vi "Initialize Tree.vi"(8 "error in":errorcluster, 10 "reference":refnum<vi>, 11 "tdms file":refnum<k34>) -> (0 "error out":errorcluster, 2 "tree reference out":refnum<vi>, 3 "tdms file out":refnum<k34>)   [LabVIEW 2019, in "Report Viewer.lvlib" / "Report Viewer.lvclass"]
uses:
  Report Viewer.lvclass
panel:
  out "Group Load":u64(slide)=38 scale=-1.0..1260.0
  out "TDMS Load":u64(slide)=38 scale=-1.0..11.0
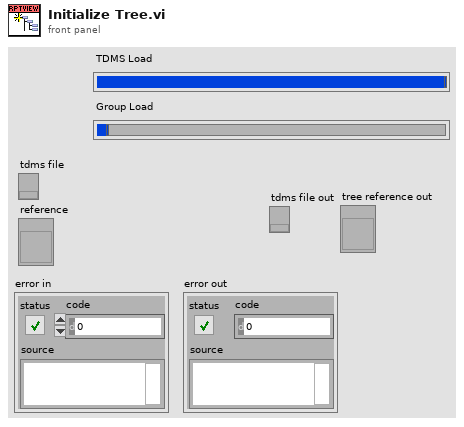
[diagram p1: front panel]
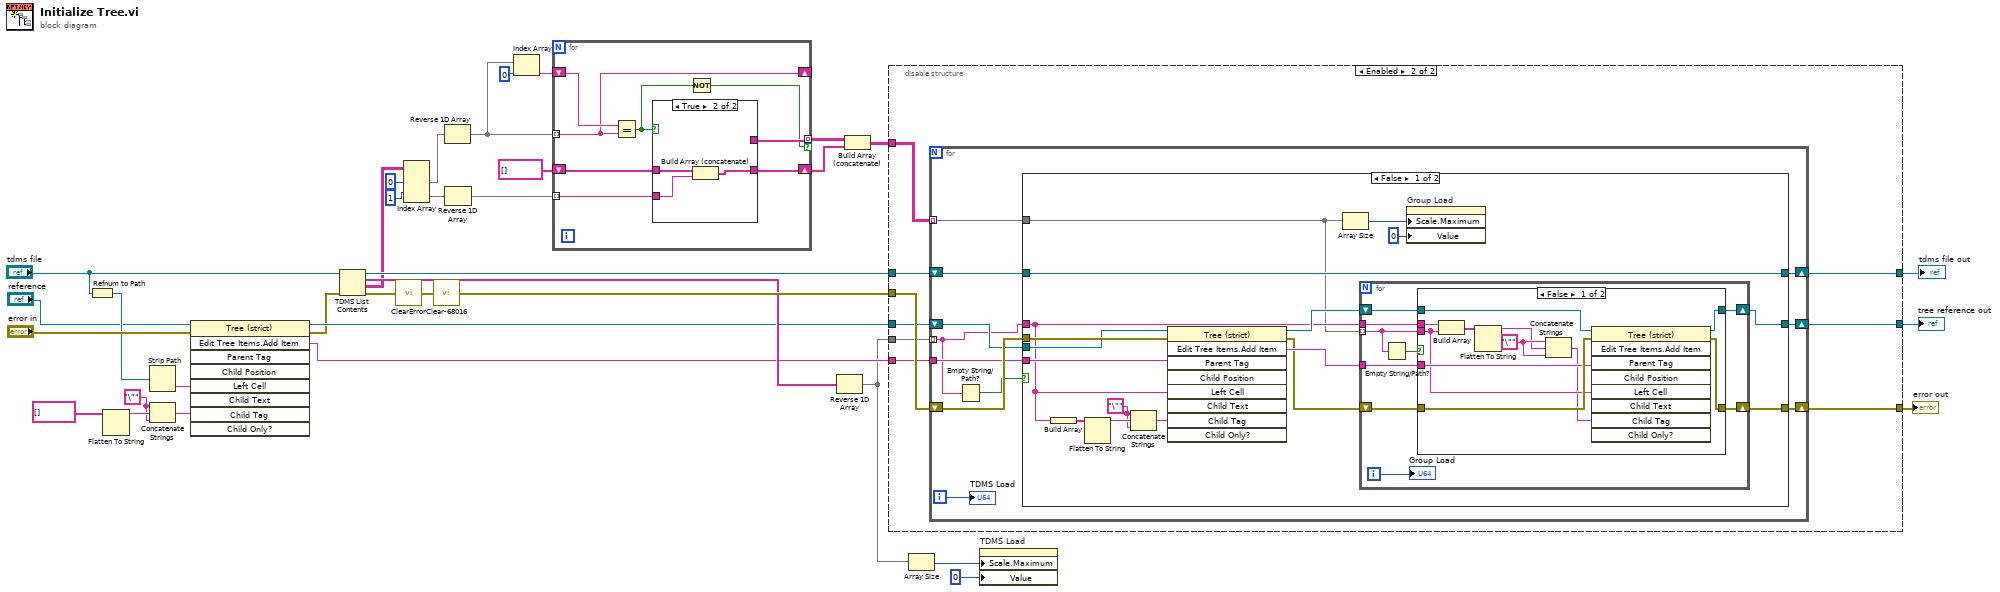
[diagram p0: block diagram]
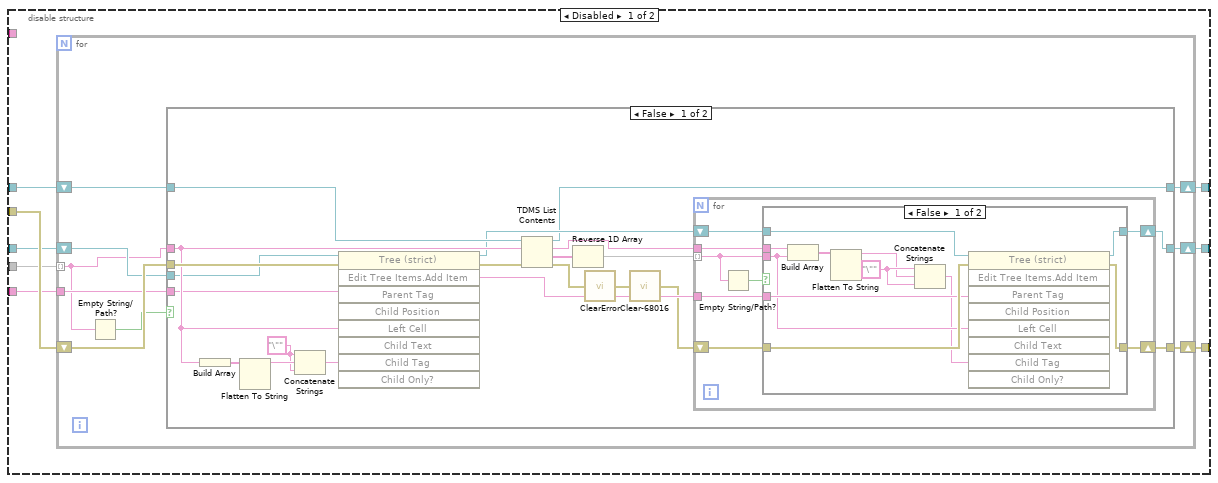
[diagram p2: hidden frame]
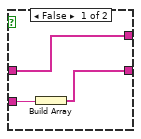
[diagram p7: hidden frame]
diagram:
  w28 = "\"" ("string")
  n1 = Refnum to Path(1:"tdms file") -> (0:w20:path)
  n2 = Flatten To String(anything=string[] [] ("appended array")) -> (data string=w29:string)  [unwired: 3 in, 2 out]
  n3 = Strip Path(path=w20) -> (name=w27:string)  [unwired: 1 out]
  n4 = Concatenate Strings(w28, w29, w28) -> (w31:string)
  n5 = invoke on="Invoke Node" class="Tree (strict)" method="Edit Tree Items.Add Item"(reference="reference", error in="error in", "Left Cell"=w27, "Child Tag"=w31) -> (reference out=w26:refnum<vi>, error out=w25:errorcluster, "Edit Tree Items:Add Item"=w32:string)  [unwired: 5 in, 6 out]
  n6 = TDMS List Contents(4:w25, 7:"tdms file") -> (0:w36:errorcluster, 1:w14:string[][], 2:w33:string[], 3:w24:refnum<k34>)  [unwired: 1 in]
  n7 = call <vilib>:"ClearError.vi"("error in (no error)"=w36) -> ("error out"=w34:errorcluster)
  n8 = Index Array(array=w14, index (row) #1=0 ("index (row)"), index (row) #2=1 ("index (row)")) -> (element #1=w2:string[], element #2=w1:string[])  [unwired: 2 in]
  n9 = call <vilib>:"Clear-68016.vi"("error in (no error)"=w34) -> ("error out"=w35:errorcluster)
  n10 = Reverse 1D Array(array=w2) -> (reversed array=w9:string[])
  n11 = Reverse 1D Array(array=w1) -> (reversed array=w12:string[])
  n12 = Index Array(array=w9, index=0) -> (element=w10:string)
  n13 = for {
    tunnel: w9 -> [w39] mode=indexing
    shift-right: [w39] -> _
    shift-left: w10 -> [w44]
    tunnel: w12 -> [w42] mode=indexing
    shift-right: [w37] -> w7
    shift-left: string[] [] -> [w43]
    tunnel: [w41] -> w8 mode=indexing if=w38
    n14 = Equal?(x=w44, y=w39) -> (x = y?=w40:bool)
    n15 = case shown="True" w40 {
      tunnel: w43 -> [w45 w49]
      tunnel: w42 -> [w46 w50]
      tunnel: [w47 w48] -> w37
      tunnel: [w45 _] -> w41
      frame False {
        n16 = Build Array(w46) -> (w47:string[])
      }
      frame True {
        n17 = Build Array (concatenate)(w49, w50) -> (w48:string[])
      }
    }
    n18 = Not(x=w40) -> (.not. x?=w38:bool)
  }
  n19 = Reverse 1D Array(array=w33) -> (reversed array=w21:string[])
  n20 = Build Array (concatenate)(w8, w7) -> (w6:string[][])
  n21 = disable-structure shown="Enabled" {
    disable-tunnel: w35 -> [w58 w121]
    disable-tunnel: w32 -> [w57 w120]
    disable-tunnel: w26 -> [w56 w119]
    disable-tunnel: w24 -> [w55 w118]
    disable-tunnel: [w54 w117] -> w23
    disable-tunnel: w21 -> [w53 w116]
    disable-tunnel: [w52 w115] -> w19
    disable-tunnel: [w51 w114] -> w18
    disable-tunnel: w6 -> [_ w113]
    frame Disabled {
      n22 = for {
        tunnel: w53 -> [w61] mode=indexing
        shift-right: [w64] -> w52
        shift-left: w55 -> [w66]
        shift-right: [w65] -> w54
        shift-left: w58 -> [w67]
        tunnel: w57 -> [w62]
        shift-right: [w59] -> w51
        shift-left: w56 -> [w63]
        n23 = Empty String/Path?(string/path=w61) -> (empty?=w60:bool)
        n24 = case shown="False" w60 {
          tunnel: w67 -> [w88 w111]
          tunnel: w66 -> [w86 w112]
          tunnel: [w85 w111] -> w65
          tunnel: [w70 w112] -> w64
          tunnel: w61 -> [w83 _]
          tunnel: w63 -> [w78 w110]
          tunnel: w62 -> [w76 _]
          tunnel: [w71 w110] -> w59
          frame False {
            w79 = "\"" ("string")
            n25 = Build Array(w83) -> (w82:string[])
            n26 = Flatten To String(anything=w82) -> (data string=w81:string)  [unwired: 3 in, 2 out]
            n27 = Concatenate Strings(w79, w81, w79) -> (w80:string)
            n28 = invoke on="Invoke Node" class="Tree (strict)" method="Edit Tree Items.Add Item"(reference=w78, error in=w88, "Parent Tag"=w76, "Left Cell"=w83, "Child Tag"=w80) -> (reference out=w77:refnum<vi>, error out=w87:errorcluster, "Edit Tree Items:Add Item"=w84:string)  [unwired: 4 in, 6 out]
            n29 = TDMS List Contents(4:w87, 6:w83, 7:w86) -> (0:w72:errorcluster, 1:w75:string[], 2:w69:string, 3:w70:refnum<k34>)
            n30 = Reverse 1D Array(array=w75) -> (reversed array=w68:string[])
            n31 = call <vilib>:"ClearError.vi"("error in (no error)"=w72) -> ("error out"=w74:errorcluster)
            n32 = call <vilib>:"Clear-68016.vi"("error in (no error)"=w74) -> ("error out"=w73:errorcluster)
            n33 = for {
              tunnel: w68 -> [w91] mode=indexing
              shift-right: [w95] -> w85
              shift-left: w73 -> [w96]
              tunnel: w84 -> [w94]
              tunnel: w69 -> [w93]
              shift-right: [w89] -> w71
              shift-left: w77 -> [w90]
              n34 = Empty String/Path?(string/path=w91) -> (empty?=w92:bool)
              n35 = case shown="False" w92 {
                tunnel: w96 -> [w107 w109]
                tunnel: [w106 w109] -> w95
                tunnel: w94 -> [w105 _]
                tunnel: w91 -> [w103 _]
                tunnel: w93 -> [w102 _]
                tunnel: w90 -> [w98 w108]
                tunnel: [w97 w108] -> w89
                frame False {
                  w101 = "\"" ("string")
                  n36 = Build Array(w102, w103) -> (w104:string[])
                  n37 = Flatten To String(anything=w104) -> (data string=w99:string)  [unwired: 3 in, 2 out]
                  n38 = Concatenate Strings(w101, w99, w101) -> (w100:string)
                  n39 = invoke on="Invoke Node" class="Tree (strict)" method="Edit Tree Items.Add Item"(reference=w98, error in=w107, "Parent Tag"=w105, "Left Cell"=w103, "Child Tag"=w100) -> (reference out=w97:refnum<vi>, error out=w106:errorcluster)  [unwired: 4 in, 7 out]
                }
                frame True {
                }
              }
            }
          }
          frame True {
          }
        }
      }
    }
    frame Enabled {
      n40 = for {
        tunnel: w116 -> [w126] mode=indexing
        shift-right: [w129] -> w115
        shift-left: w118 -> [w131]
        shift-right: [w130] -> w117
        shift-left: w121 -> [w132]
        tunnel: w120 -> [w127]
        shift-right: [w124] -> w114
        shift-left: w119 -> [w128]
        tunnel: w113 -> [w123] mode=indexing
        i -> [w122]
        n41 = Empty String/Path?(string/path=w126) -> (empty?=w125:bool)
        n42 = case shown="False" w125 {
          tunnel: w132 -> [w149 w173]
          tunnel: w131 -> [w136 w174]
          tunnel: [w148 w173] -> w130
          tunnel: [w136 w174] -> w129
          tunnel: w126 -> [w138 _]
          tunnel: w128 -> [w142 w172]
          tunnel: w127 -> [w140 _]
          tunnel: [w139 w172] -> w124
          tunnel: w123 -> [w134 _]
          frame False {
            w143 = "\"" ("string")
            n43 = Build Array(w138) -> (w146:string[])
            n44 = Flatten To String(anything=w146) -> (data string=w145:string)  [unwired: 3 in, 2 out]
            n45 = Concatenate Strings(w143, w145, w143) -> (w144:string)
            n46 = invoke on="Invoke Node" class="Tree (strict)" method="Edit Tree Items.Add Item"(reference=w142, error in=w149, "Parent Tag"=w140, "Left Cell"=w138, "Child Tag"=w144) -> (reference out=w141:refnum<vi>, error out=w137:errorcluster, "Edit Tree Items:Add Item"=w147:string)  [unwired: 4 in, 6 out]
            n47 = Array Size(array=w134) -> (size(s)=w133:i32)
            n48 = for {
              tunnel: w134 -> [w153] mode=indexing
              shift-right: [w157] -> w148
              shift-left: w137 -> [w158]
              tunnel: w147 -> [w156]
              tunnel: w138 -> [w155]
              shift-right: [w151] -> w139
              shift-left: w141 -> [w152]
              i -> [w150]
              n49 = Empty String/Path?(string/path=w153) -> (empty?=w154:bool)
              n50 = case shown="False" w154 {
                tunnel: w158 -> [w169 w171]
                tunnel: [w168 w171] -> w157
                tunnel: w156 -> [w167 _]
                tunnel: w153 -> [w165 _]
                tunnel: w155 -> [w164 _]
                tunnel: w152 -> [w160 w170]
                tunnel: [w159 w170] -> w151
                frame False {
                  w163 = "\"" ("string")
                  n51 = Build Array(w164, w165) -> (w166:string[])
                  n52 = Flatten To String(anything=w166) -> (data string=w161:string)  [unwired: 3 in, 2 out]
                  n53 = Concatenate Strings(w163, w161, w163) -> (w162:string)
                  n54 = invoke on="Invoke Node" class="Tree (strict)" method="Edit Tree Items.Add Item"(reference=w160, error in=w169, "Parent Tag"=w167, "Left Cell"=w165, "Child Tag"=w162) -> (reference out=w159:refnum<vi>, error out=w168:errorcluster)  [unwired: 4 in, 7 out]
                }
                frame True {
                }
              }
              "Group Load" <- w150
            }
            n55 = property on="Group Load" class="Slide (strict)"("Scale.Maximum"=w133, "Value"=u64 0 ("Group Load")) -> ()  [unwired: 2 in, 2 out]
          }
          frame True {
          }
        }
        "TDMS Load" <- w122
      }
    }
  }
  "error out" <- w23
  "tdms file out" <- w19
  "tree reference out" <- w18
  n56 = Array Size(array=w21) -> (size(s)=w4:i32)
  n57 = property on="TDMS Load" class="Slide (strict)"("Scale.Maximum"=w4, "Value"=u8 0 ("TDMS FILE IS LOADING")) -> ()  [unwired: 2 in, 2 out]
